vi "GetTriggerOutputEvents.vi"(8 "Error In":errorcluster, 11 "Keithley 6482 In":refnum<visa-resource-name>) -> (0 "Error Out":errorcluster, 2 "Trigger Events":enum16{"Source", "Delay", "Sense", "None"}[](array[ring]), 3 "Keithley 6482 Out":refnum<visa-resource-name>)   [LabVIEW 2012, in "Keithley-6482.lvlib"]
uses:
  Keithley-6482.lvlib
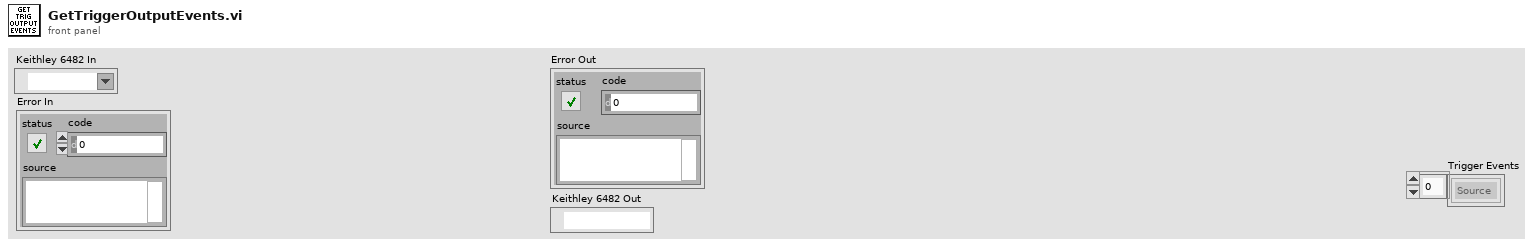
[diagram p1: front panel]
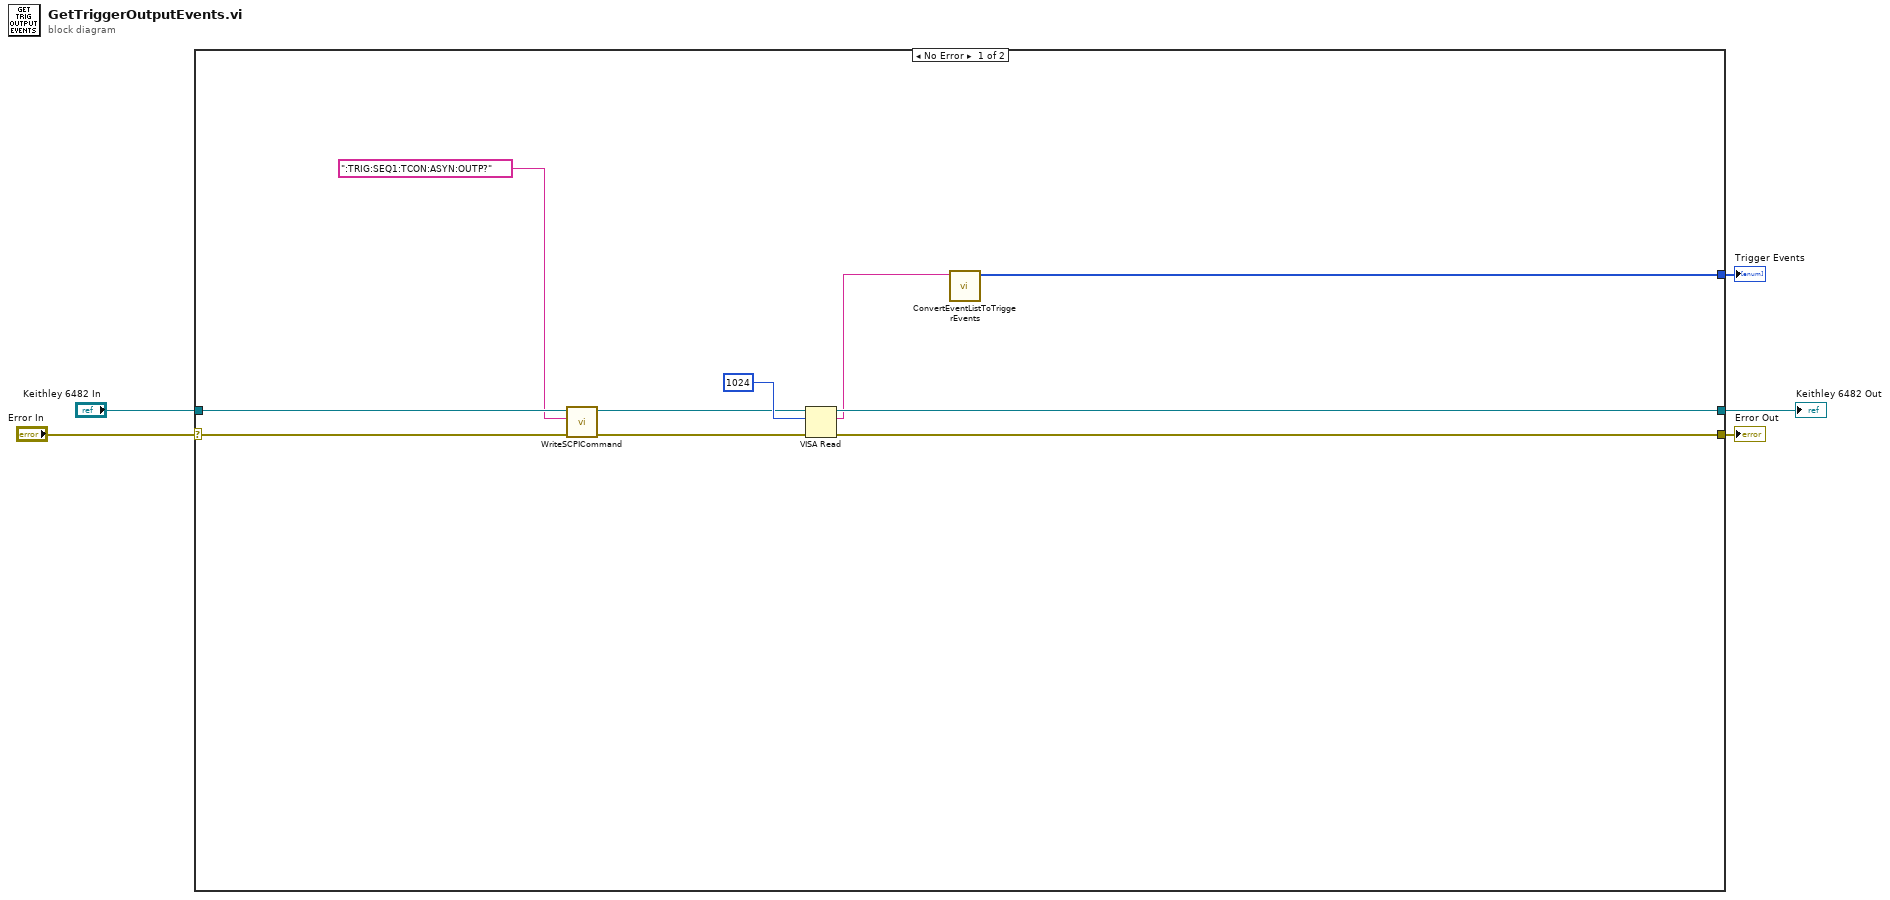
[diagram p0: block diagram]
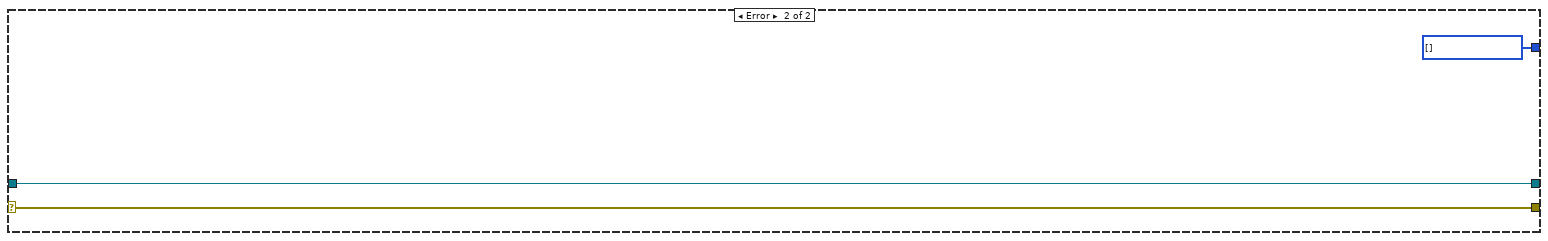
[diagram p2: hidden frame]
diagram:
  n1 = case shown="No Error" "Error In" {
    selector: "Error In" -> [w10 w17]
    tunnel: "Keithley 6482 In" -> [w9 w18]
    tunnel: [w15 w17] -> w3
    tunnel: [w14 w18] -> w2
    tunnel: [w6 w16] -> w1
    frame No Error {
      n2 = call "WriteSCPICommand.vi"("Error In"=w10, "SCPI Command"=":TRIG:SEQ1:TCON:ASYN:OUTP?", "Keithley 6482 In"=w9) -> ("Error Out"=w11:errorcluster, "Keithley 6482 Out"=w12:refnum<visa-resource-name>)  [unwired: 7 in]
      n3 = VISA Read(VISA resource name=w12, byte count=u32 1024, error in (no error)=w11) -> (VISA resource name out=w14:refnum<visa-resource-name>, read buffer=w7:string, error out=w15:errorcluster)  [unwired: 1 out]
      n4 = call "ConvertEventListToTriggerEvents.vi"("Event List"=w7) -> ("Trigger Events"=w6:enum16{"Source", "Delay", "Sense", "None"}[])  [unwired: 10 in]
    }
    frame Error {
      w16 = enum16{"Source", "Delay", "Sense", "None"}[] [] items=["Source", "Delay", "Sense", "None"] ("Trigger Events")
    }
  }
  "Error Out" <- w3
  "Keithley 6482 Out" <- w2
  "Trigger Events" <- w1
